vi "OpenCV-FaceDetectMask.vi"() -> ()   [LabVIEW 2017]
uses:
  IMAQCV/IMAQCV.lvlib
  IMAQCV/LVOpenCV.lvlib
panel:
  in  "type":enum16{"GRAY", "COLOR"}(ring)=enum."COLOR"
  in  "Image Size":T1(ring)
  out "picture":picture
  in  "Mask picture path":path=path "c:/vision/masks/2.jpg"
  in  "stop":bool
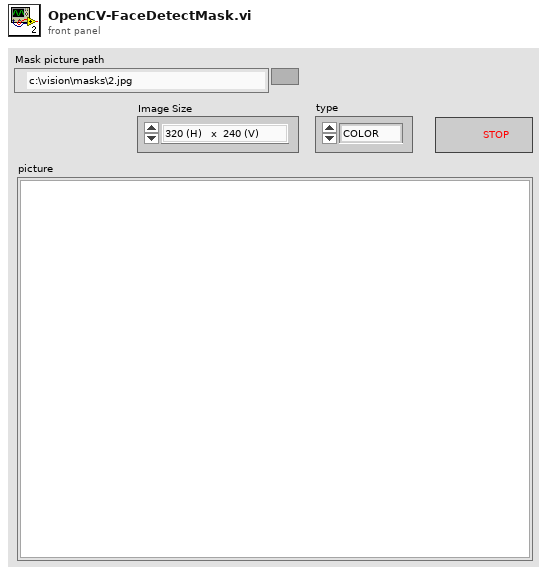
[diagram p1: front panel]
types:
  T1 = enum16{"320 (H)   x  240 (V)", "352(H)    x  288 (V)", "640 (H)   x  480 (V) ", "800 (H)   x  600 (V)", "1024 (H) x  768 (V)", "1280 (H) x  720 (V)", "1280 (H) x  960 (V)", "1280 (H) x 1024 (V)", "1920 (H) x 1080 (V)"}
  T2 = typedef "IMAQCV.lvlib/IMAQCV Image.ctl" = refnum<vi>
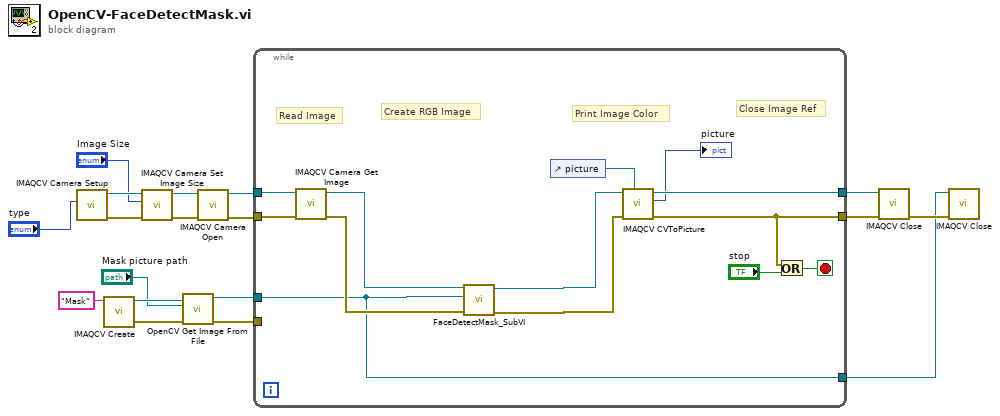
[diagram p0: block diagram]
diagram:
  n1 = call "IMAQCV Camera Setup.vi"("type"="type") -> ("error out"=w10:errorcluster, "image out"=w9:T2)  [unwired: 9 in]
  n2 = call "IMAQCV Create.vi"("Image Name"="Mask") -> ("error out"=w17:errorcluster, "Image Out"=w16:T2)  [unwired: 9 in]
  n3 = call "IMAQCV Camera Set Image Size.vi"("error in (no error)"=w10, "Image Size"="Image Size", "image in"=w9) -> ("error out"=w11:errorcluster, "image out"=w8:T2)  [unwired: 7 in]
  n4 = call "OpenCV Get Image From File.vi"("error in (no error)"=w17, "path"="Mask picture path", "CVImage"=w16) -> ("error out"=w3:errorcluster, "Image Out"=w4:T2)  [unwired: 7 in]
  n5 = call "IMAQCV Camera Open.vi"("error in (no error)"=w11, "image in"=w8) -> ("error out"=w12:errorcluster, "image out"=w7:T2)  [unwired: 8 in]
  n6 = while {
    tunnel: w7 -> [w30]
    tunnel: [w29] -> w13
    tunnel: w12 -> [w31]
    tunnel: [w20] -> w14
    tunnel: w4 -> [w19]
    tunnel: w3 -> [_]
    tunnel: [w19] -> w1
    stop <- w21 stop-if-true
    # "Print Image Color"
    # "Close Image Ref"
    # "Create RGB Image"
    # "Read Image"
    n7 = call "IMAQCV Camera Get Image.vi"("error in (no error)"=w31, "image in"=w30) -> ("error out"=w25:errorcluster, "image out"=w24:T2)  [unwired: 8 in]
    n8 = call "FaceDetectMask_SubVI.vi"("error in (no error)"=w25, "mask"=w19, "image"=w24) -> ("error out"=w27:errorcluster, "image out"=w26:T2)  [unwired: 7 in]
    n9 = control-ref of="picture"() -> (w23:refnum<vi>)
    n10 = call "IMAQCV CVToPicture.vi"("picture ref"=w23, "error in (no error)"=w27, "image"=w26) -> ("error out"=w20:errorcluster, "picture"=→"picture":picture, "image out"=w29:T2)  [unwired: 6 in]
    n11 = Or(x=w20, y="stop") -> (x .or. y?=w21:bool)
  }
  n12 = call "IMAQCV Close.vi"("error in (no error)"=w14, "Image"=w13) -> ("error out"=w2:errorcluster)  [unwired: 9 in]
  n13 = call "IMAQCV Close.vi"("error in (no error)"=w2, "Image"=w1) -> ()  [unwired: 9 in, 1 out]
